vi "Reset.vi"(8 "error in (no error)":errorcluster, 10 "target time(1s)":dbl=1.0, 11 "Timer in":refnum<class "Timer.lvclass">) -> (0 "error out":errorcluster, 3 "Timer out":refnum<class "Timer.lvclass">)   [LabVIEW 2020, in "Timer.lvclass"]
uses:
  Timer.lvclass
  Timer.lvclass/Timer.ctl
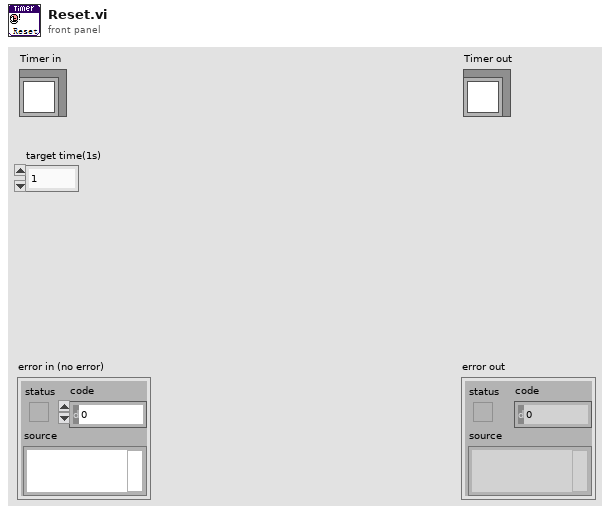
[diagram p1: front panel]
types:
  T1 = cluster{"target time(ms)":u32, "elapsed time(ms)":u32, "start time":u32, "pause":bool, "auto reset":bool}
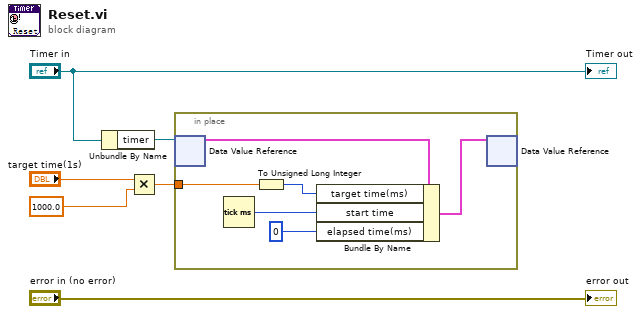
[diagram p0: block diagram]
diagram:
  n1 = Unbundle By Name("Timer in") -> ("timer"=w4:refnum<data-value>)
  n2 = Multiply(x="target time(1s)", y=1000.0) -> (x*y=w1:dbl)
  n3 = in-place {
    in-place-border: w1 -> [w7]
    n4 = in-place-dvr #1(w4) -> (w11:T1)  [unwired: 1 out]
    n5 = Tick Count (ms)() -> (millisecond timer value=w12:u32)
    n6 = To Unsigned Long Integer(number=w7) -> (unsigned 32bit integer=w9:u32)
    n7 = Bundle By Name(cluster=w11, "target time(ms)"=w9, "start time"=w12, "elapsed time(ms)"=u32 0) -> (w10:T1)
    n8 = in-place-dvr #1(w10) -> ()  [unwired: 2 out]
  }
  "error out" <- "error in (no error)"
  "Timer out" <- "Timer in"
